vi "Main Program - Torque Testing Interface.vi"() -> ()   [LabVIEW 2019]
uses:
  Serial Comms/Serial - Settings.ctl
  Controls/System State.ctl
  Controls/User Interface Cluster.ctl
  Serial Comms/Serial Connection States.ctl
  <vilib>/Utility/error.llb/DialogType.ctl
panel:
  in  "Load Settings":bool
  in  "Save Settings":bool
  in  "Shutdown":bool
  out "Mark-10 System State:":T1
  in  "Tab Control":enum32{"Setup", "Run", "Settings"}(tab)
  in  "Serial Port":refnum<visa-resource-name>
  in  "Serial Settings":T2={"baud rate"=115200, "data bits"=8, "parity"=enum."None", "stop bits"=10, "flow control"=0} {"flow control" items=["None"=0, "XON/XOFF"=1, "RTS/CTS"=2, "DTR/DSR"=4]; "stop bits" items=["1.0"=10, "1.5"=15, "2.0"=20]; "data bits" min=5 max=8 step=1; "baud rate" items=["75"=75, "110"=110, "134"=134, "150"=150, "300"=300, "600"=600, "1200"=1200, "1800"=1800, "2400"=2400, "4800"=4800, "7200"=7200, "9600"=9600, "14400"=14400, "19200"=19200, "28800"=28800, "38400"=38400, "56000"=56000, "57600"=57600, "115200"=115200, "128000"=128000, "230400"=230400]}
  in  "Connect":bool
  in  "Turn to Zero Position":bool
  in  "Sample Number:":u32
  in  "Sample Prefix:":string="Applicator Test"
  in  "Generate Filepath":bool
  in  "Set Zero Position":bool
  in  "Stop Button":bool
  in  "Start Test":bool
  in  "Winding Speed":dbl=20.0 format="%.2f°/s"
  in  "Winding Distance":dbl=296.0 format="%.2f°"
  out "XY Graph":cluster{"Y":dbl[], "Y":dbl[]}(graph)
  in  "Output Data Path":path
  in  "Settings File Path":path=path "C:/Users/Public/Data/Mark-10-Settings.ini"
  in  "Output Data Base Path":path=path "C:/Users/Public/Data"
  in  "Auto-Increment Sample Number":bool=TRUE
  # "Winding (CW)"
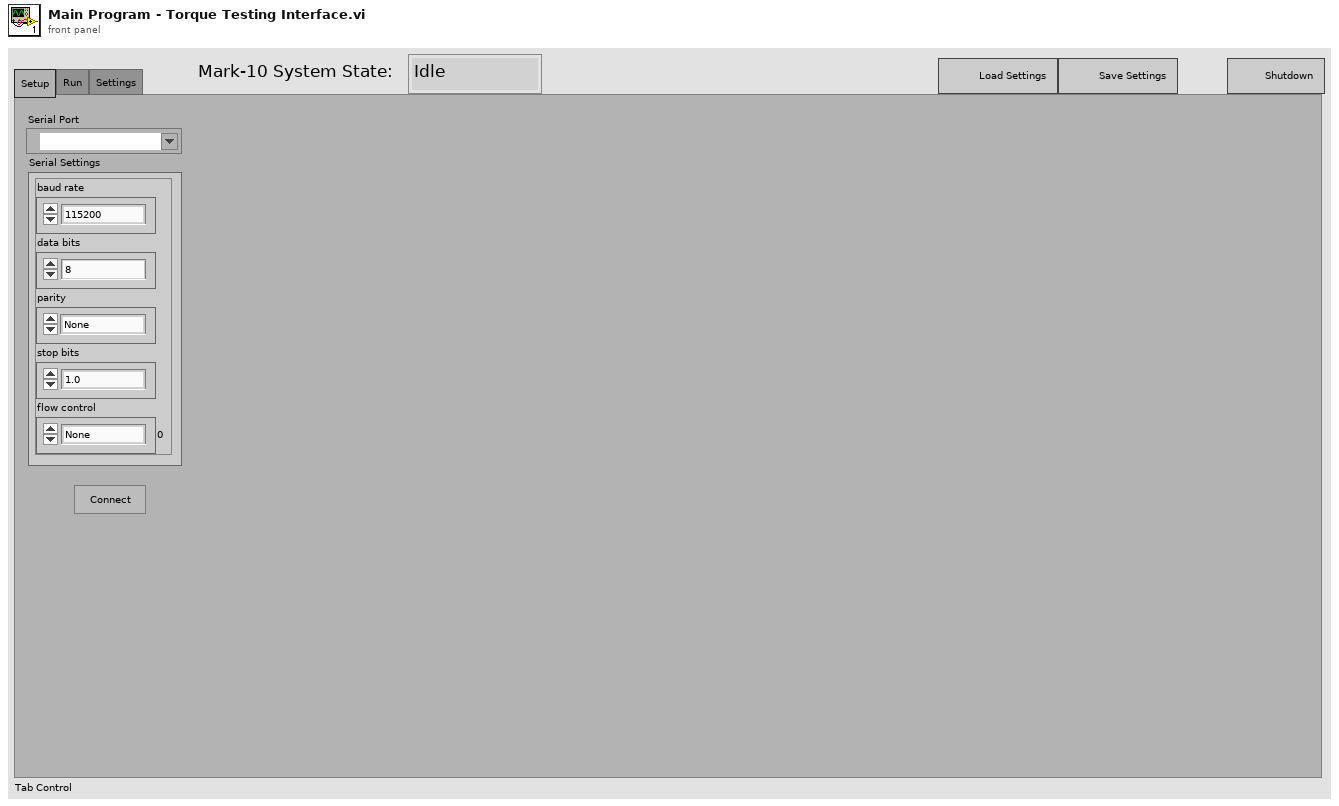
[diagram p1: front panel]
types:
  T1 = typedef "System State.ctl" = enum16{"Idle", "Initialize", "Testing", "Stop", "Shutdown"}
  T2 = typedef "Serial - Settings.ctl" = cluster{"baud rate":u32, "data bits":u16, "parity":enum16{"None", "Odd", "Even", "Mark", "Space"}, "stop bits":u16, "flow control":u16}
  T3 = typedef "User Interface Cluster.ctl" = cluster{"Serial Settings":T2, "Serial Port":refnum<visa-resource-name>, "Winding Distance (degrees)":dbl, "Winding Speed":dbl, "Dwell time (s)":dbl, "Unwinding Distance (degrees)":dbl, "Unwinding Speed":dbl, "Output Data Path":path, "Sample Prefix:":string, "Sample Number:":u32, "Output Data Base Path":path, "Auto-Increment Sample Number":bool}
  T4 = typedef "Serial Connection States.ctl" = enum16{"Connect", "Get Connection", "Disconnect"}
  T5 = typedef "DialogType.ctl" = u16
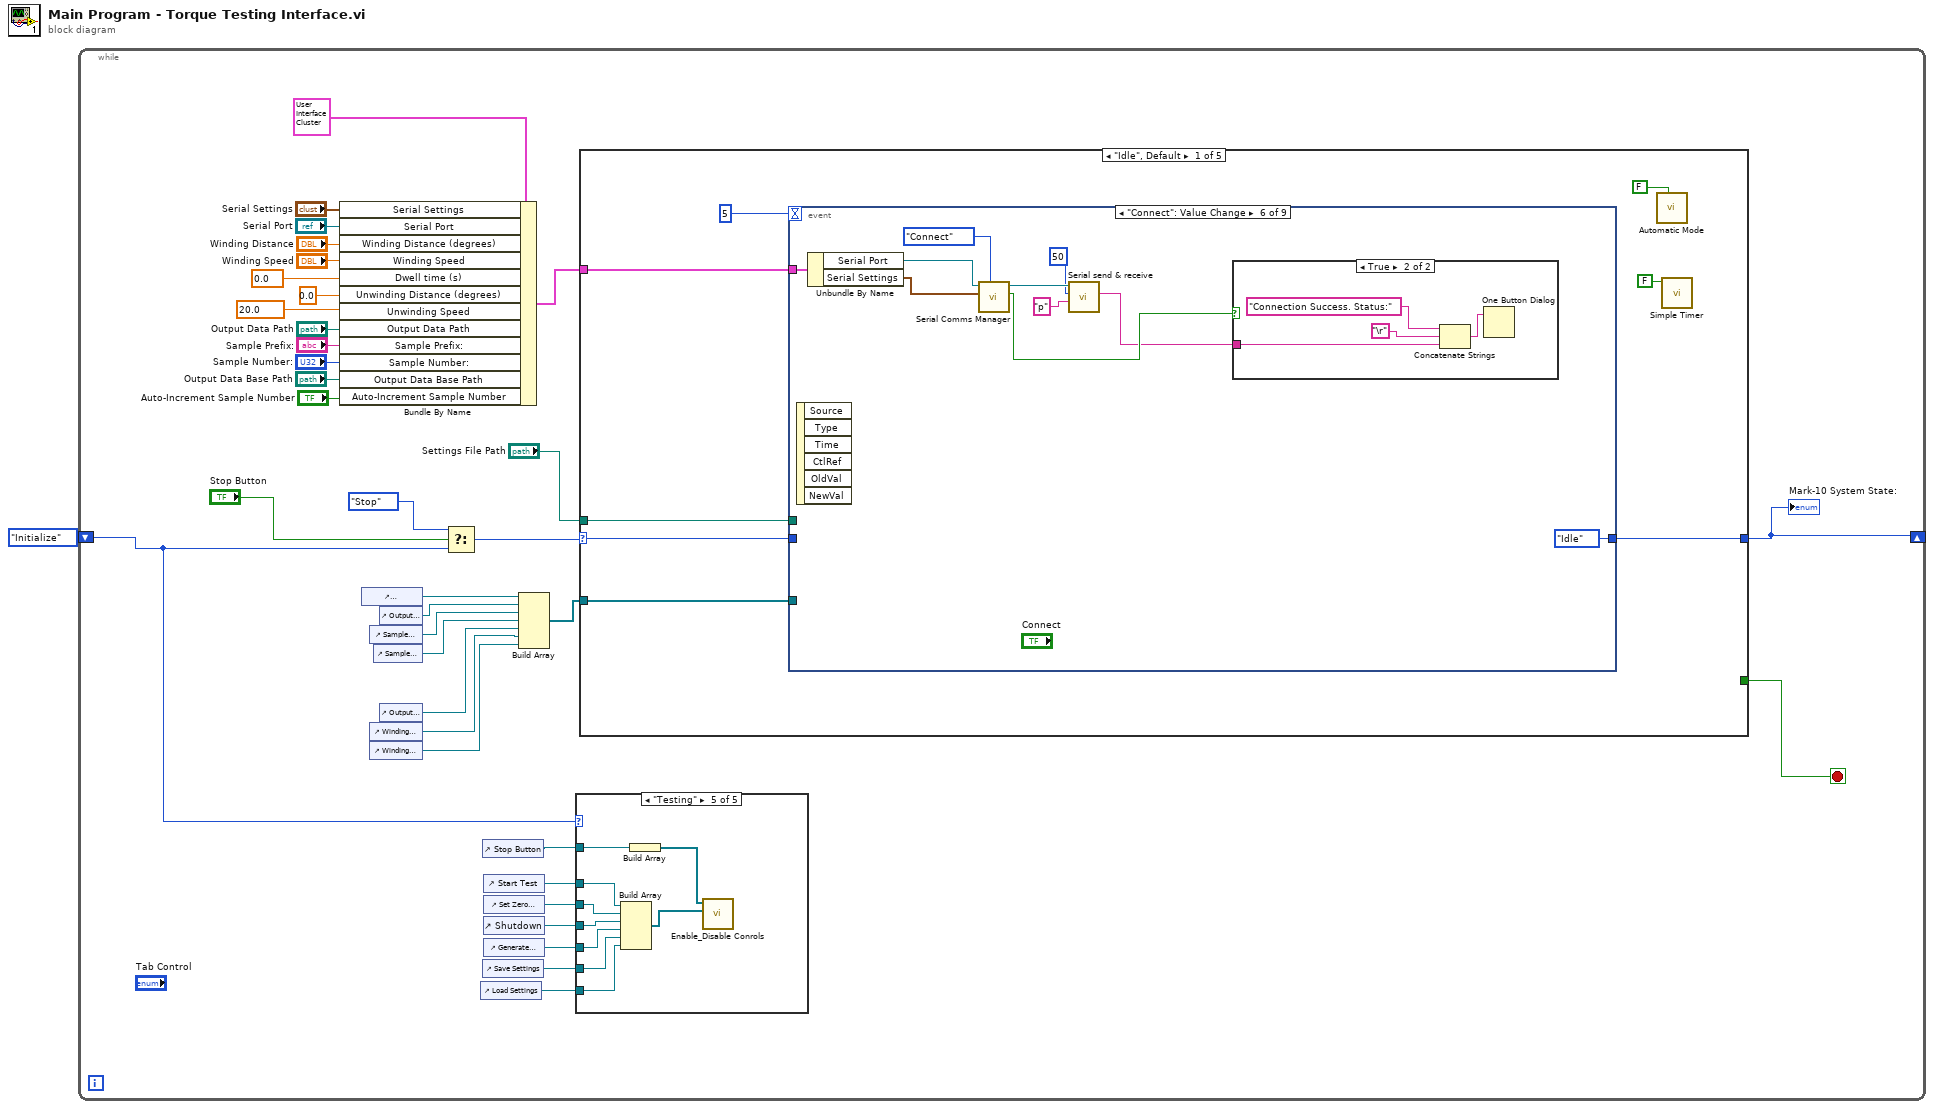
[diagram p0: block diagram]
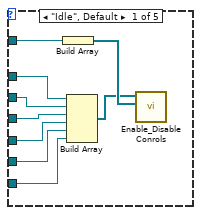
[diagram p2: hidden frame]
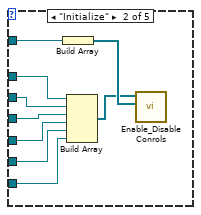
[diagram p3: hidden frame]
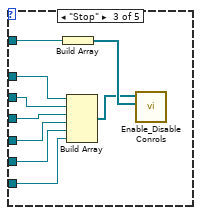
[diagram p4: hidden frame]
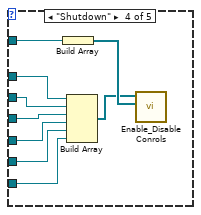
[diagram p5: hidden frame]
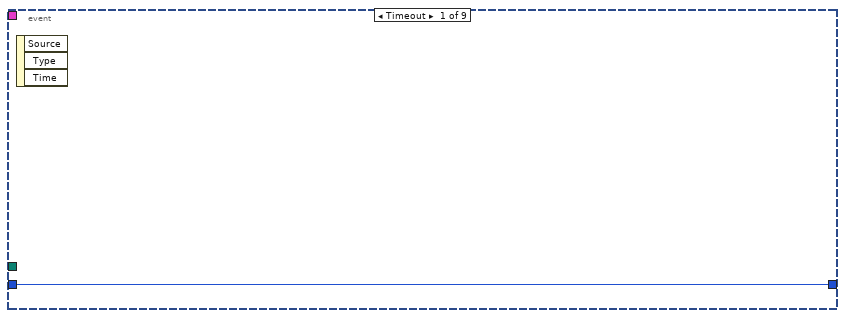
[diagram p6: hidden frame]
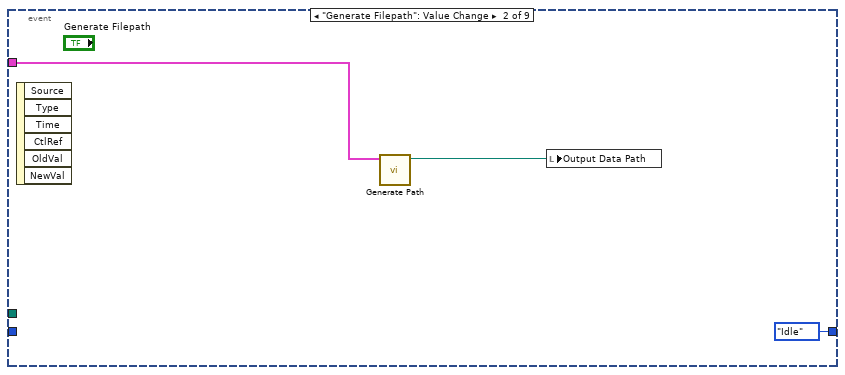
[diagram p7: hidden frame]
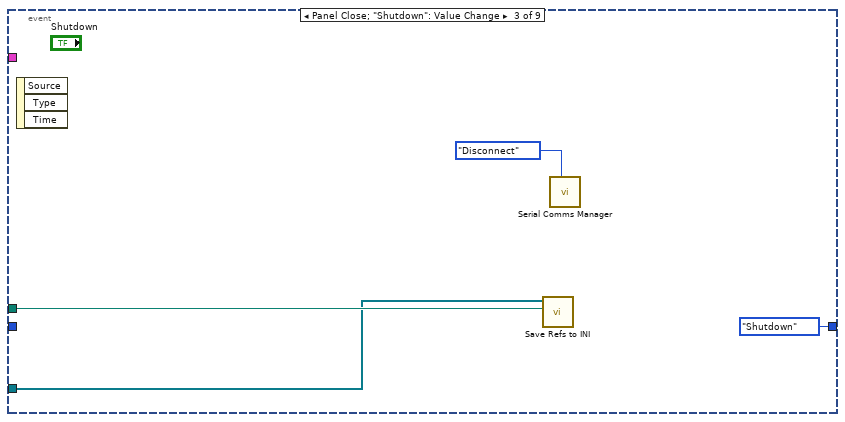
[diagram p8: hidden frame]
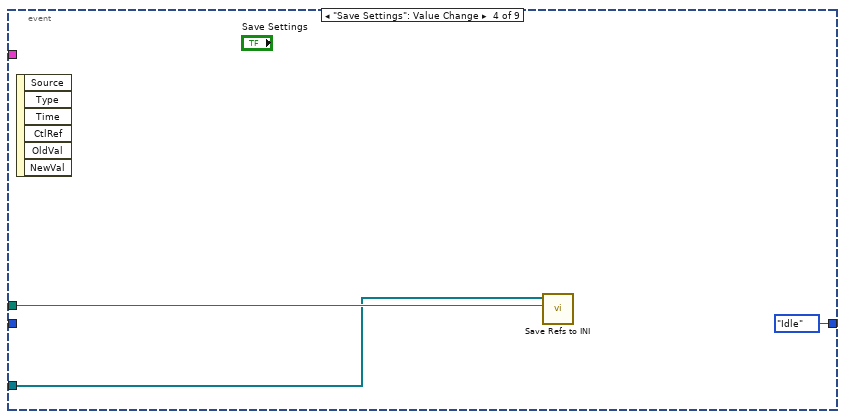
[diagram p9: hidden frame]
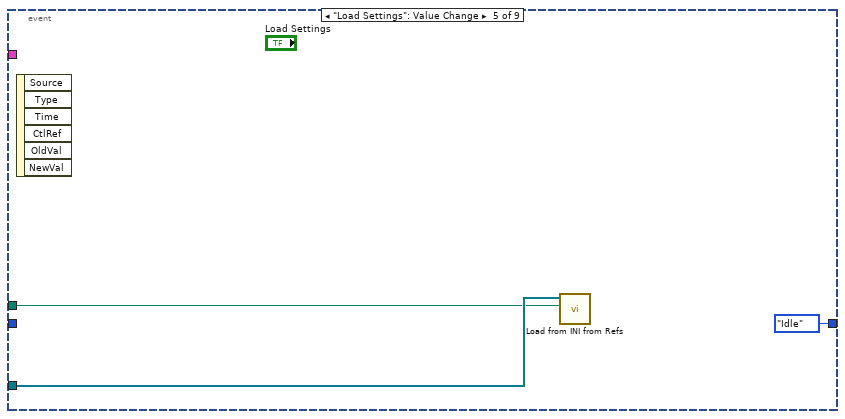
[diagram p10: hidden frame]
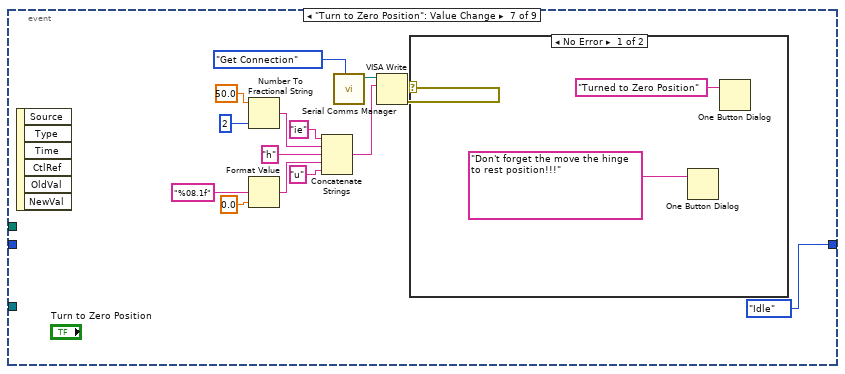
[diagram p12: hidden frame]
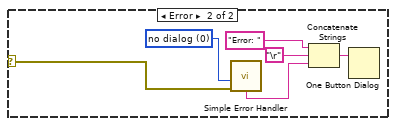
[diagram p13: hidden frame]
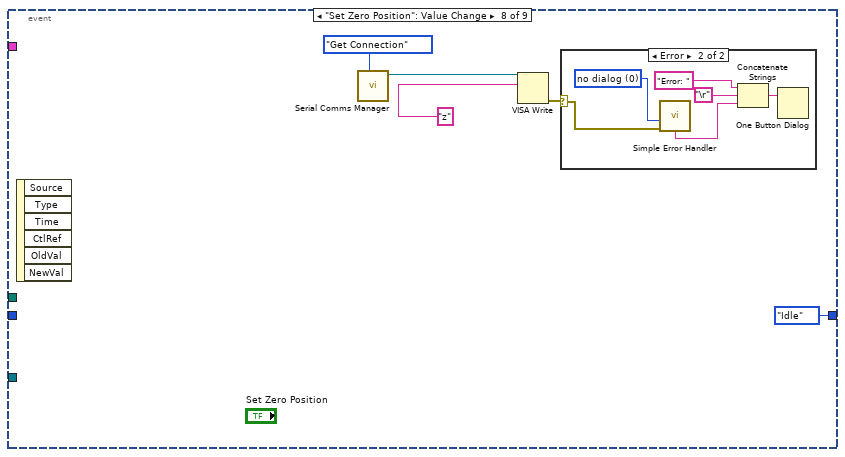
[diagram p14: hidden frame]
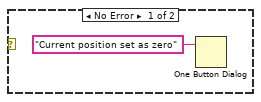
[diagram p15: hidden frame]
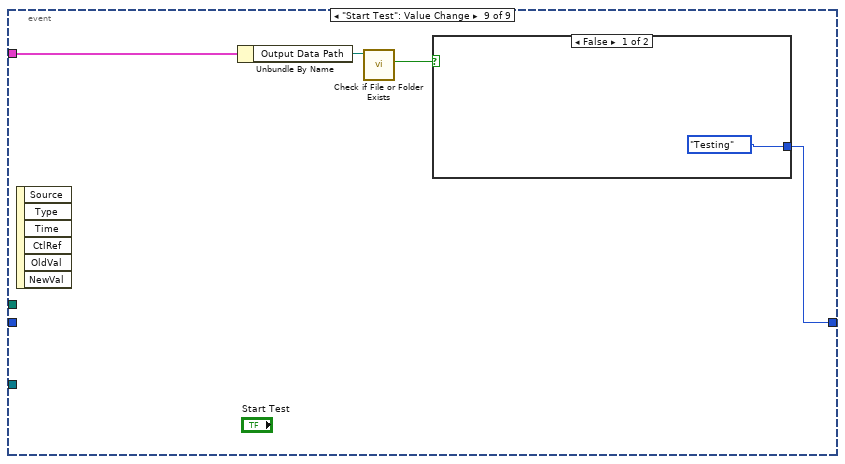
[diagram p16: hidden frame]
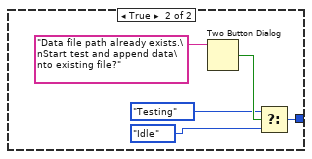
[diagram p17: hidden frame]
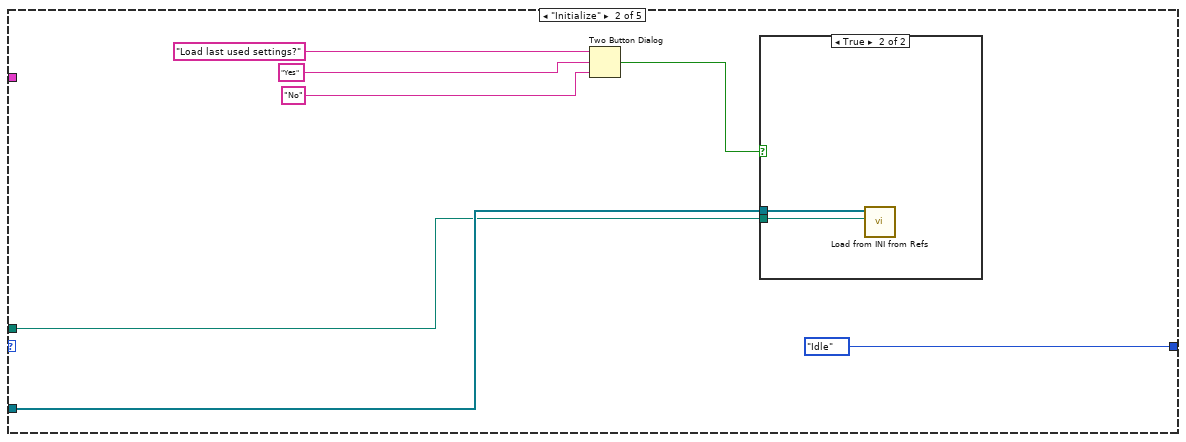
[diagram p18: hidden frame]
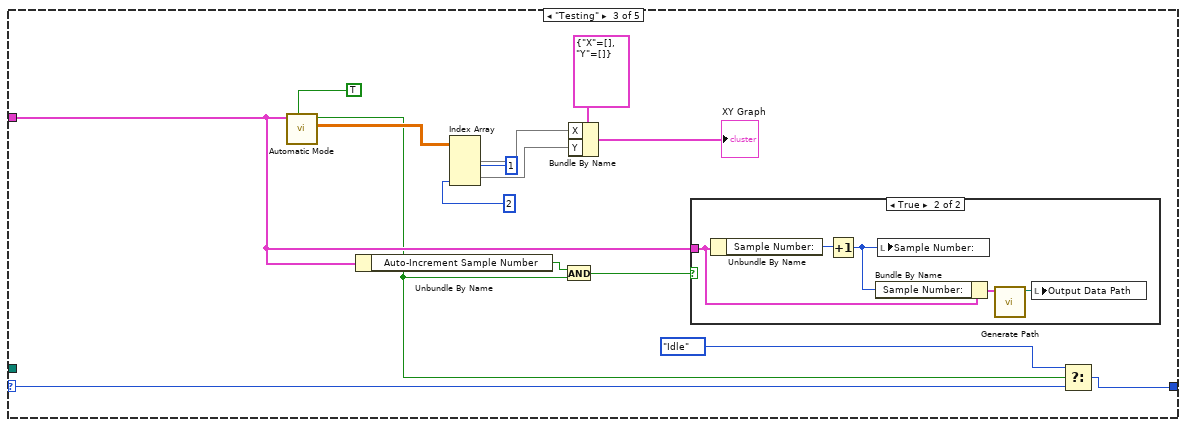
[diagram p20: hidden frame]
diagram:
  n1 = while {
    shift-right: [w37] -> _
    shift-left: System_State."Initialize" -> [w7]
    stop <- w14 stop-if-true
    n2 = Bundle By Name(cluster=T3 {"Serial Settings"={"baud rate"=9600, "data bits"=8, "parity"=enum."None", "stop bits"=10, "flow control"=0}, "Serial Port"="", "Winding Distance (degrees)"=0.0, "Winding Speed"=0.0, "Dwell time (s)"=0.0, "Unwinding Distance (degrees)"=0.0, "Unwinding Speed"=0.0, "Output Data Path"=path "", "Sample Prefix:"="Applicator Test", "Sample Number:"=0, "Output Data Base Path"=path "C:/Users/Public/Data", "Auto-Increment Sample Number"=FALSE} ("User Interface Cluster"), "Serial Settings"="Serial Settings", "Serial Port"="Serial Port", "Winding Distance (degrees)"="Winding Distance", "Winding Speed"="Winding Speed", "Dwell time (s)"=0.0, "Unwinding Distance (degrees)"=0.0, "Unwinding Speed"=20.0, "Output Data Path"="Output Data Path", "Sample Prefix:"="Sample Prefix:", "Sample Number:"="Sample Number:", "Output Data Base Path"="Output Data Base Path", "Auto-Increment Sample Number"="Auto-Increment Sample Number") -> (w28:T3)
    n3 = control-ref of="Auto-Increment Sample Number"() -> (w19:refnum<vi>)
    n4 = control-ref of="Sample Number:"() -> (w17:refnum<vi>)
    n5 = control-ref of="Winding Speed"() -> (w3:refnum<vi>)
    n6 = control-ref of="Winding Distance"() -> (w2:refnum<vi>)
    n7 = control-ref of="Sample Prefix:"() -> (w16:refnum<vi>)
    n8 = control-ref of="Output Data Base Path"() -> (w18:refnum<vi>)
    n9 = control-ref of="Output Data Path"() -> (w4:refnum<vi>)
    n10 = Select(t=System_State."Stop", s="Stop Button", f=w7) -> (s? t:f=w27:T1)
    n11 = control-ref of="Load Settings"() -> (w5:refnum<vi>)
    n12 = control-ref of="Stop Button"() -> (w8:refnum<vi>)
    n13 = control-ref of="Save Settings"() -> (w6:refnum<vi>)
    n14 = control-ref of="Start Test"() -> (w12:refnum<vi>)
    n15 = control-ref of="Set Zero Position"() -> (w11:refnum<vi>)
    n16 = control-ref of="Shutdown"() -> (w10:refnum<vi>)
    n17 = control-ref of="Generate Filepath"() -> (w9:refnum<vi>)
    n18 = Build Array(w19, w18, w17, w16, w4, w3, w2) -> (w15:refnum<vi>[])
    n19 = case shown="\"Testing\"" w7 {
      tunnel: w12 -> [w44 w53 w62 w71 w82]
      tunnel: w11 -> [w43 w52 w61 w70 w81]
      tunnel: w10 -> [w42 w51 w60 w69 w80]
      tunnel: w9 -> [w41 w50 w59 w68 w79]
      tunnel: w8 -> [w40 w49 w58 w67 w78]
      tunnel: w6 -> [w39 w48 w57 w66 w75]
      tunnel: w5 -> [w38 w47 w56 w65 w74]
      frame "Idle", Default {
        n20 = Build Array(w40) -> (w46:refnum<vi>[])
        n21 = Build Array(w44, w43, w42, w41, w39, w38) -> (w45:refnum<vi>[])
        n22 = call "Enable_Disable Conrols.vi"("Controls to Disable"=w46, "Controls to Enable"=w45) -> ()  [unwired: 10 in]
      }
      frame "Initialize" {
        n23 = Build Array(w49) -> (w55:refnum<vi>[])
        n24 = Build Array(w53, w52, w51, w50, w48, w47) -> (w54:refnum<vi>[])
        n25 = call "Enable_Disable Conrols.vi"("Controls to Disable"=w55, "Controls to Enable"=w54) -> ()  [unwired: 10 in]
      }
      frame "Stop" {
        n26 = Build Array(w58) -> (w64:refnum<vi>[])
        n27 = Build Array(w62, w61, w60, w59, w57, w56) -> (w63:refnum<vi>[])
        n28 = call "Enable_Disable Conrols.vi"("Controls to Disable"=w64, "Controls to Enable"=w63) -> ()  [unwired: 10 in]
      }
      frame "Shutdown" {
        n29 = Build Array(w67) -> (w73:refnum<vi>[])
        n30 = Build Array(w71, w70, w69, w68, w66, w65) -> (w72:refnum<vi>[])
        n31 = call "Enable_Disable Conrols.vi"("Controls to Disable"=w73, "Controls to Enable"=w72) -> ()  [unwired: 10 in]
      }
      frame "Testing" {
        n32 = Build Array(w82, w81, w80, w79, w75, w74) -> (w77:refnum<vi>[])
        n33 = Build Array(w78) -> (w76:refnum<vi>[])
        n34 = call "Enable_Disable Conrols.vi"("Controls to Disable"=w77, "Controls to Enable"=w76) -> ()  [unwired: 10 in]
      }
    }
    n35 = case shown="\"Idle\", Default" w27 {
      selector: w27 -> [w89 _ w185 _ _]
      tunnel: [w88 System_State."Idle" w184 System_State."Idle" System_State."Shutdown"] -> w37
      tunnel: w28 -> [w87 _ w175 _ _]
      tunnel: "Settings File Path" -> [w84 w163 _ _ _]
      tunnel: w15 -> [w83 w164 _ _ _]
      tunnel: [_ _ _ _ TRUE] -> w14
      frame "Idle", Default {
        n36 = event shown="[5] \"Connect\": Value Change" {
          selector: _ -> [_ _ _ _ _ _ _ _ _]
          dyn-events: _ -> [_ _ _ _ _ _ _ _ _]
          timeout: 5 -> [_ _ _ _ _ _ _ _ _]
          tunnel: w89 -> [w91 _ _ _ _ _ _ _ _]
          tunnel: [w91 System_State."Idle" System_State."Shutdown" System_State."Idle" System_State."Idle" System_State."Idle" System_State."Idle" System_State."Idle" w153] -> w88
          tunnel: w87 -> [_ w94 _ _ _ w113 _ _ w156]
          tunnel: w84 -> [_ _ w96 w100 w103 _ _ _ _]
          tunnel: w83 -> [_ _ w95 w99 w104 _ _ _ _]
          event Timeout {
            n37 = event-data() -> ()  [unwired: 1 in, 3 out]
          }
          event "Generate Filepath": Value Change {
            n38 = event-data() -> ()  [unwired: 1 in, 6 out]
            n39 = call "Generate Path.vi"("User Interface Cluster"=w94) -> ("appended path"=w93:path)  [unwired: 10 in]
            n40 = local write "Output Data Path"(w93) -> ()
          }
          event Panel Close; "Shutdown": Value Change {
            n41 = event-data() -> ()  [unwired: 1 in, 3 out]
            n42 = call "Save Refs to INI.vi"("Configuration file path"=w96, "Array of Control References"=w95) -> ()  [unwired: 10 in]
            n43 = call "Serial Comms Manager.vi"("Action"=Serial_Connection_States."Disconnect") -> ()  [unwired: 9 in, 2 out]
          }
          event "Save Settings": Value Change {
            n44 = event-data() -> ()  [unwired: 1 in, 6 out]
            n45 = call "Save Refs to INI.vi"("Configuration file path"=w100, "Array of Control References"=w99) -> ()  [unwired: 10 in]
          }
          event "Load Settings": Value Change {
            n46 = event-data() -> ()  [unwired: 1 in, 6 out]
            n47 = call "Load from INI from Refs.vi"("Configuration file path"=w103, "Array of Control References"=w104) -> ()  [unwired: 10 in]
          }
          event "Connect": Value Change {
            n48 = event-data() -> ()  [unwired: 1 in, 6 out]
            n49 = Unbundle By Name(w113) -> ("Serial Port"=w112:refnum<visa-resource-name>, "Serial Settings"=w111:T2)
            n50 = call "Serial Comms Manager.vi"("Action"=Serial_Connection_States."Connect", "Serial Settings"=w111, "VISA Refnum in"=w112) -> ("Success?"=w108:bool, "VISA resource name out"=w109:refnum<visa-resource-name>)  [unwired: 7 in]
            n51 = call "Serial send & receive.vi"("Command"="p", "delay before read (ms)"=u32 50, "VISA Refnum in"=w109) -> ("read buffer"=w105:string)  [unwired: 7 in, 1 out]
            n52 = case shown="True" w108 {
              tunnel: w105 -> [_ w116]
              frame False {
              }
              frame True {
                n53 = Concatenate Strings("Connection Success. Status:" ("message"), "\r", w116) -> (w115:string)
                n54 = One Button Dialog(message=w115) -> ()  [unwired: 1 in, 1 out]
              }
            }
          }
          event "Turn to Zero Position": Value Change {
            n55 = event-data() -> ()  [unwired: 1 in, 6 out]
            n56 = Number To Fractional String(number=50.0, precision (6)=i16 2) -> (F-format string=w129:string)  [unwired: 2 in]
            n57 = Format Value(format string="%08.1f", value (0)=0.0) -> (output string=w126:string)  [unwired: 1 in]
            n58 = Concatenate Strings("ie", w129, "h" ("string"), w126, "u" ("string")) -> (w124:string)
            n59 = call "Serial Comms Manager.vi"("Action"=Serial_Connection_States."Get Connection") -> ("VISA resource name out"=w131:refnum<visa-resource-name>)  [unwired: 9 in, 1 out]
            n60 = VISA Write(VISA resource name=w131, write buffer=w124) -> (error out=w120:errorcluster)  [unwired: 1 in, 2 out]
            n61 = case shown="No Error" w120 {
              selector: w120 -> [_ w139]
              frame No Error {
                n62 = One Button Dialog(message="Don't forget the move the hinge to rest position!!!") -> ()  [unwired: 1 in, 1 out]
                n63 = One Button Dialog(message="Turned to Zero Position") -> ()  [unwired: 1 in, 1 out]
              }
              frame Error {
                w140 = T5 0 items=["no dialog", "OK message", "continue or stop message", "OK message + warnings", "continue/stop + warnings"] ("type of dialog (OK msg:1)")
                n64 = call <vilib>:"Simple Error Handler.vi"("type of dialog (OK msg:1)"=w140, "error in (no error)"=w139) -> ("message"=w135:string)  [unwired: 3 in, 4 out]
                n65 = Concatenate Strings("Error: ", "\r", w135) -> (w136:string)
                n66 = One Button Dialog(message=w136) -> ()  [unwired: 1 in, 1 out]
              }
            }
          }
          event "Set Zero Position": Value Change {
            n67 = event-data() -> ()  [unwired: 1 in, 6 out]
            n68 = call "Serial Comms Manager.vi"("Action"=Serial_Connection_States."Get Connection") -> ("VISA resource name out"=w144:refnum<visa-resource-name>)  [unwired: 9 in, 1 out]
            n69 = VISA Write(VISA resource name=w144, write buffer="z") -> (error out=w141:errorcluster)  [unwired: 1 in, 2 out]
            n70 = case shown="Error" w141 {
              selector: w141 -> [_ w151]
              frame No Error {
                n71 = One Button Dialog(message="Current position set as zero") -> ()  [unwired: 1 in, 1 out]
              }
              frame Error {
                w152 = T5 0 items=["no dialog", "OK message", "continue or stop message", "OK message + warnings", "continue/stop + warnings"] ("type of dialog (OK msg:1)")
                n72 = call <vilib>:"Simple Error Handler.vi"("type of dialog (OK msg:1)"=w152, "error in (no error)"=w151) -> ("message"=w147:string)  [unwired: 3 in, 4 out]
                n73 = Concatenate Strings("Error: ", "\r", w147) -> (w148:string)
                n74 = One Button Dialog(message=w148) -> ()  [unwired: 1 in, 1 out]
              }
            }
          }
          event "Start Test": Value Change {
            n75 = event-data() -> ()  [unwired: 1 in, 6 out]
            n76 = Unbundle By Name(w156) -> ("Output Data Path"=w155:path)
            n77 = call <vilib>:"Check if File or Folder Exists.vi"("path"=w155) -> ("file or folder exists?"=w154:bool)  [unwired: 8 in, 2 out]
            n78 = case shown="False" w154 {
              tunnel: [System_State."Testing" w158] -> w153
              frame False {
              }
              frame True {
                n79 = Two Button Dialog(message="Data file path already exists.\nStart test and append data\nto existing file?") -> (T button?=w161:bool)  [unwired: 2 in]
                n80 = Select(t=System_State."Testing", s=w161, f=System_State."Idle") -> (s? t:f=w158:T1)
              }
            }
          }
        }
        n81 = call "Automatic Mode.vi"("Testing"=FALSE) -> ()  [unwired: 9 in, 2 out]
        n82 = call "Simple Timer.vi"("Timing?"=FALSE) -> ()  [unwired: 9 in, 2 out]
      }
      frame "Initialize" {
        n83 = Two Button Dialog(message="Load last used settings?", 1:"No" ("F button name (\"Cancel\")"), 2:"Yes" ("T button name (\"OK\")")) -> (T button?=w165:bool)
        n84 = case shown="True" w165 {
          tunnel: w164 -> [_ w171]
          tunnel: w163 -> [_ w170]
          frame False {
          }
          frame True {
            n85 = call "Load from INI from Refs.vi"("Configuration file path"=w170, "Array of Control References"=w171) -> ()  [unwired: 10 in]
          }
        }
      }
      frame "Testing" {
        n86 = call "Automatic Mode.vi"("Testing"=TRUE, "User Interface Cluster"=w175) -> ("Output Data"=w182:dbl[][], "Test Complete"=w173:bool)  [unwired: 8 in]
        n87 = Unbundle By Name(w175) -> ("Auto-Increment Sample Number"=w174:bool)
        n88 = Index Array(array=w182, index (col) #1=1 ("disabled index (col)"), index (col) #2=2 ("index (col)")) -> (element #1=w178:dbl[], element #2=w177:dbl[])  [unwired: 2 in]
        n89 = And(x=w174, y=w173) -> (x .and. y?=w172:bool)
        n90 = Bundle By Name(cluster=cluster{"X":dbl[], "Y":dbl[]} {"X"=[], "Y"=[]}, "X"=w178, "Y"=w177) -> (→"XY Graph":cluster{"X":dbl[], "Y":dbl[]})
        n91 = case shown="True" w172 {
          tunnel: w175 -> [_ w190]
          frame False {
          }
          frame True {
            n92 = Unbundle By Name(w190) -> ("Sample Number:"=w191:u32)
            n93 = Increment(x=w191) -> (x+1=w189:u32)
            n94 = Bundle By Name(cluster=w190, "Sample Number:"=w189) -> (w188:T3)
            n95 = local write "Sample Number:"(w189) -> ()
            n96 = call "Generate Path.vi"("User Interface Cluster"=w188) -> ("appended path"=w187:path)  [unwired: 10 in]
            n97 = local write "Output Data Path"(w187) -> ()
          }
        }
        n98 = Select(t=System_State."Idle", s=w173, f=w185) -> (s? t:f=w184:T1)
      }
      frame "Stop" {
        n99 = call "Serial Comms Manager.vi"("Action"=Serial_Connection_States."Get Connection") -> ("VISA resource name out"=w194:refnum<visa-resource-name>)  [unwired: 9 in, 1 out]
        n100 = VISA Write(VISA resource name=w194, write buffer="s") -> (error out=w192:errorcluster)  [unwired: 1 in, 2 out]
        n101 = case shown="Error" w192 {
          selector: w192 -> [_ w201]
          frame No Error {
          }
          frame Error {
            w202 = T5 0 items=["no dialog", "OK message", "continue or stop message", "OK message + warnings", "continue/stop + warnings"] ("type of dialog (OK msg:1)")
            n102 = call <vilib>:"Simple Error Handler.vi"("type of dialog (OK msg:1)"=w202, "error in (no error)"=w201) -> ("message"=w197:string)  [unwired: 3 in, 4 out]
            n103 = Concatenate Strings("Error: ", "\r", w197) -> (w198:string)
            n104 = One Button Dialog(message=w198) -> ()  [unwired: 1 in, 1 out]
          }
        }
      }
      frame "Shutdown" {
      }
    }
    "Mark-10 System State:" <- w37
  }
